vi "write_image_XYscan.vi"() -> ()   [LabVIEW 2011]
panel:
  out "chanel num":u8
  in  "chan_num":u8
  out "Position num":u8
  out "Chemin":path
  in  "Pos_num":u8
  in  "Chemin 2":path
  out "Imtemp":u16[][](array[numeric])
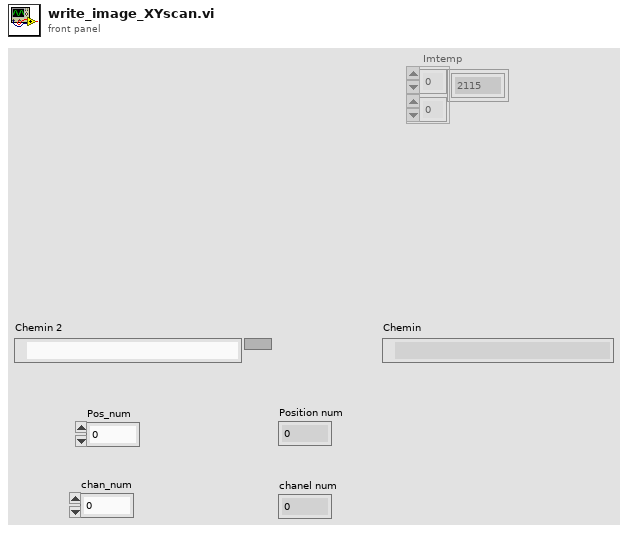
[diagram p1: front panel]
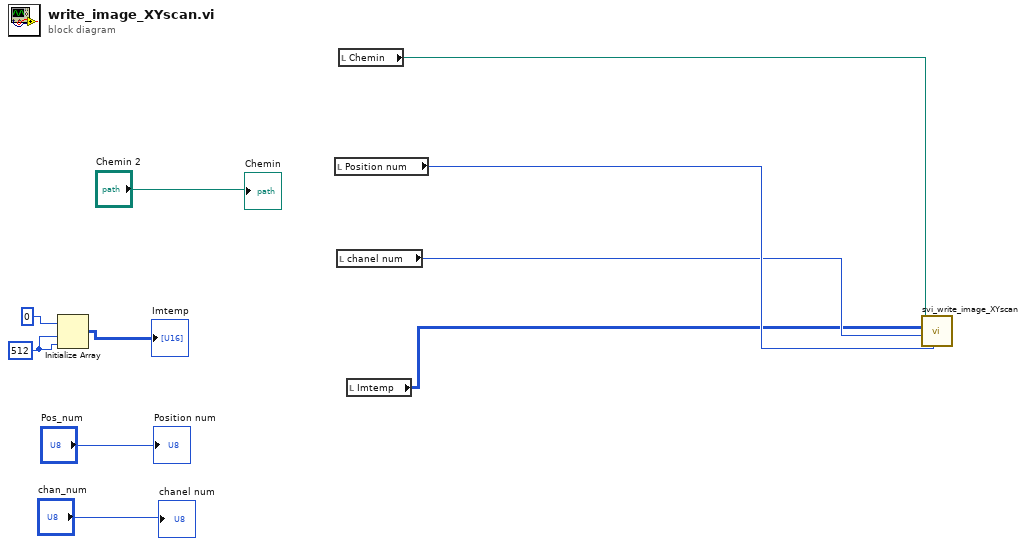
[diagram p0: block diagram]
diagram:
  w8 = 512
  n1 = Initialize Array(u16 0, w8, w8) -> (→"Imtemp":u16[][])
  n2 = local read "Position num"() -> (w3:u8)
  n3 = local read "chanel num"() -> (w2:u8)
  n4 = local read "Chemin"() -> (w4:path)
  n5 = local read "Imtemp"() -> (w1:u16[][])
  n6 = call "svi_write_image_XYscan.vi"("Position num"=w3, "chanel num"=w2, "image in"=w1, "Chemin"=w4) -> ()  [unwired: 8 in]
  "Chemin" <- "Chemin 2"
  "Position num" <- "Pos_num"
  "chanel num" <- "chan_num"
